vi "FPGA_Check_Pins_target.vi"() -> ()   [LabVIEW 2018]
uses:
  <vilib>/Platform/TimedLoop/XDataNode/timing_clust.ctl
  <vilib>/Platform/TimedLoop/XDataNode/nitl_modes.ctl
  <vilib>/Platform/TimedLoop/XDataNode/wakeup.ctl
  <vilib>/rvi/Emulation/niFpgaGetClockAttributes.vi
  <vilib>/rvi/Emulation/niFpgaSctlEmulationGetInTimedLoop.vi
  <vilib>/rvi/Emulation/niFpgaEmulationReportErrorSimple.vi
  <vilib>/rvi/eio/common/nirviEmuTemplateMethod_errors.vi
  <vilib>/rvi/Emulation/niFpgaCriticalErrorInLSC.vi
  <vilib>/rvi/Emulation/niFpgaProcessEmulError.vi
  <vilib>/eio/EIONode/EIONode.xnode
  <vilib>/Platform/TimedLoop/XDataNode/XDataNode.xnode
  <vilib>/Platform/TimedLoop/XDataNode/XDNodeRunTimeDep.lvlib
panel:
  out "Delay B to A":i16
  out "Delay A to B":i16
  out "Operation compl":bool
  out "DDCB_PFI3_Read":bool
  out "DDCB_PFI2_Read":bool
  out "DDCB_PFI1_Read":bool
  out "DDCA_PFI3_Read":bool
  out "DDCA_PFI2_Read":bool
  out "DDCA_PFI1_Read":bool
  in  "Write to PFI":u8
  in  "Cycle":bool
  out "Read Port 2 B":u8 format="%b"
  out "Read Port 1 B":u8 format="%b"
  out "Read Port 0 B":u8 format="%b"
  in  "A to B/B to A":bool
  in  "Write to":u8 format="%b"
  out "Read Port 2 A":u8 format="%b"
  out "Read Port 1 A":u8 format="%b"
  out "Read Port 0 A":u8 format="%b"
  in  "Source Freq":refnum<k21>="100 MHz Clock"
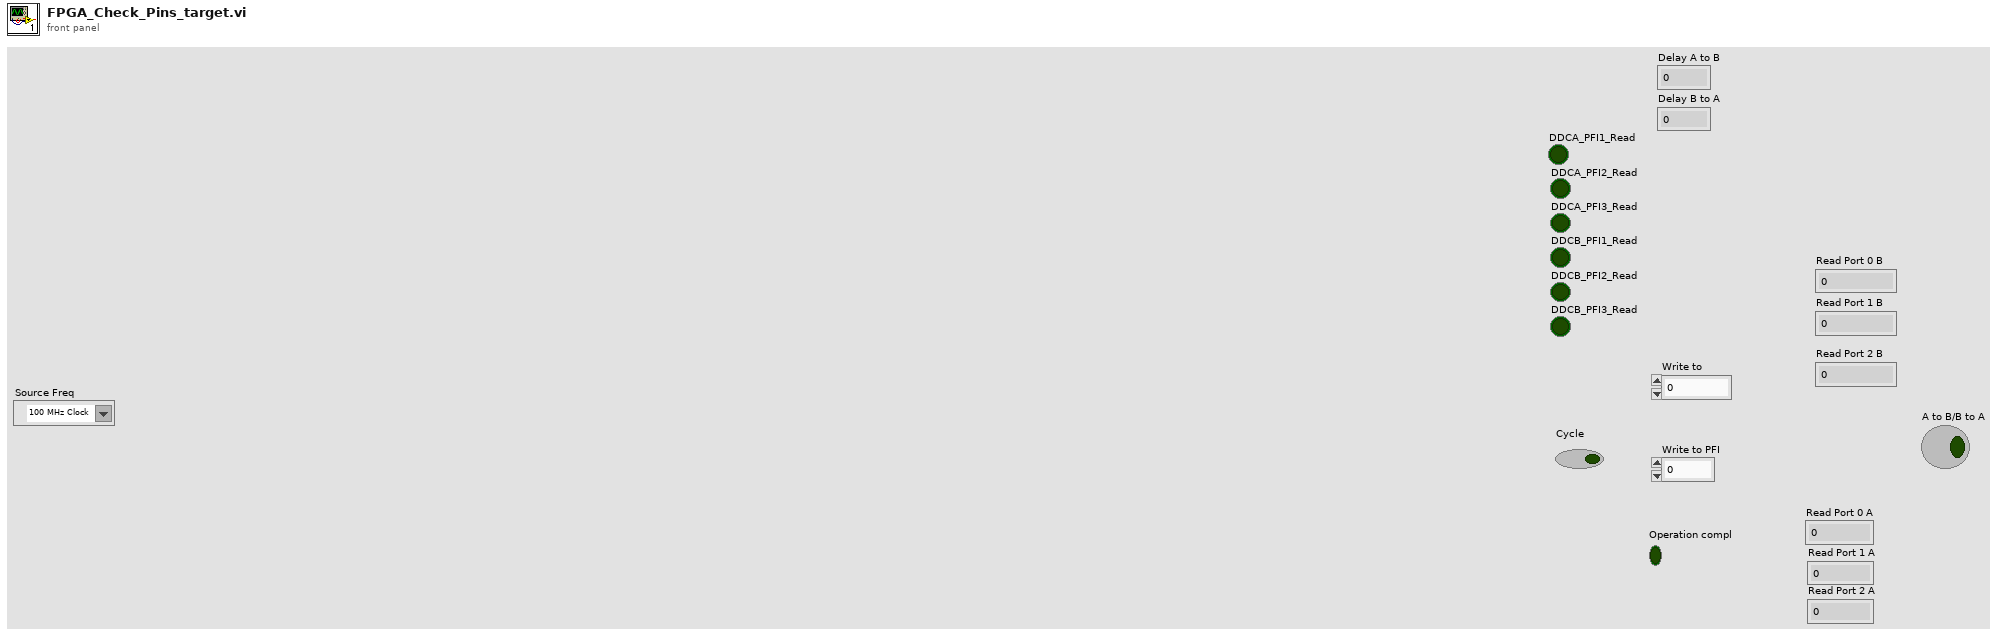
[diagram p1: front panel]
types:
  T1 = typedef "XDNodeRunTimeDep.lvlib/timing_clust.ctl" = cluster{"Expected End [f-1]":u64, "Actual End [f-1]":u64, "Finished Late? [f-1]":bool, "Expected End [i-1]":u64, "Actual End [i-1]":u64, "Finished Late? [i-1]":bool, "Expected Start [i]":u64, "Actual Start [i]":u64, "Expected Start [f]":u64, "Actual Start [f]":u64, "Source Name":string, "Structure Name":string, "Period":i64, "Deadline":i64, "Offset":i64, "Start":i64, "Priority":i32, "Timeout":i32, "Mode":T2, "Wakeup Reason":T3, "Error":errorcluster, "Source Type":string, "Secondary Source Type":string, "Global End Time":u64, "Global Start Time":u64, "Frame Duration":u64, "Iteration Duration":u64, "Assigned CPU":i32, "I/O Scan Engine Mode":u32}
  T2 = typedef "XDNodeRunTimeDep.lvlib/nitl_modes.ctl" = enum32{"No Change", "Process missed periods, maintain original phase", "Discard missed periods, maintain original phase", "Process missed periods, ignore original phase", "Discard missed periods, ignore original phase"}
  T3 = typedef "XDNodeRunTimeDep.lvlib/wakeup.ctl" = enum32{"Normal", "Aborted", "Asynchronous wakeup", "Timing source error", "Timed loop error", "Timeout"}
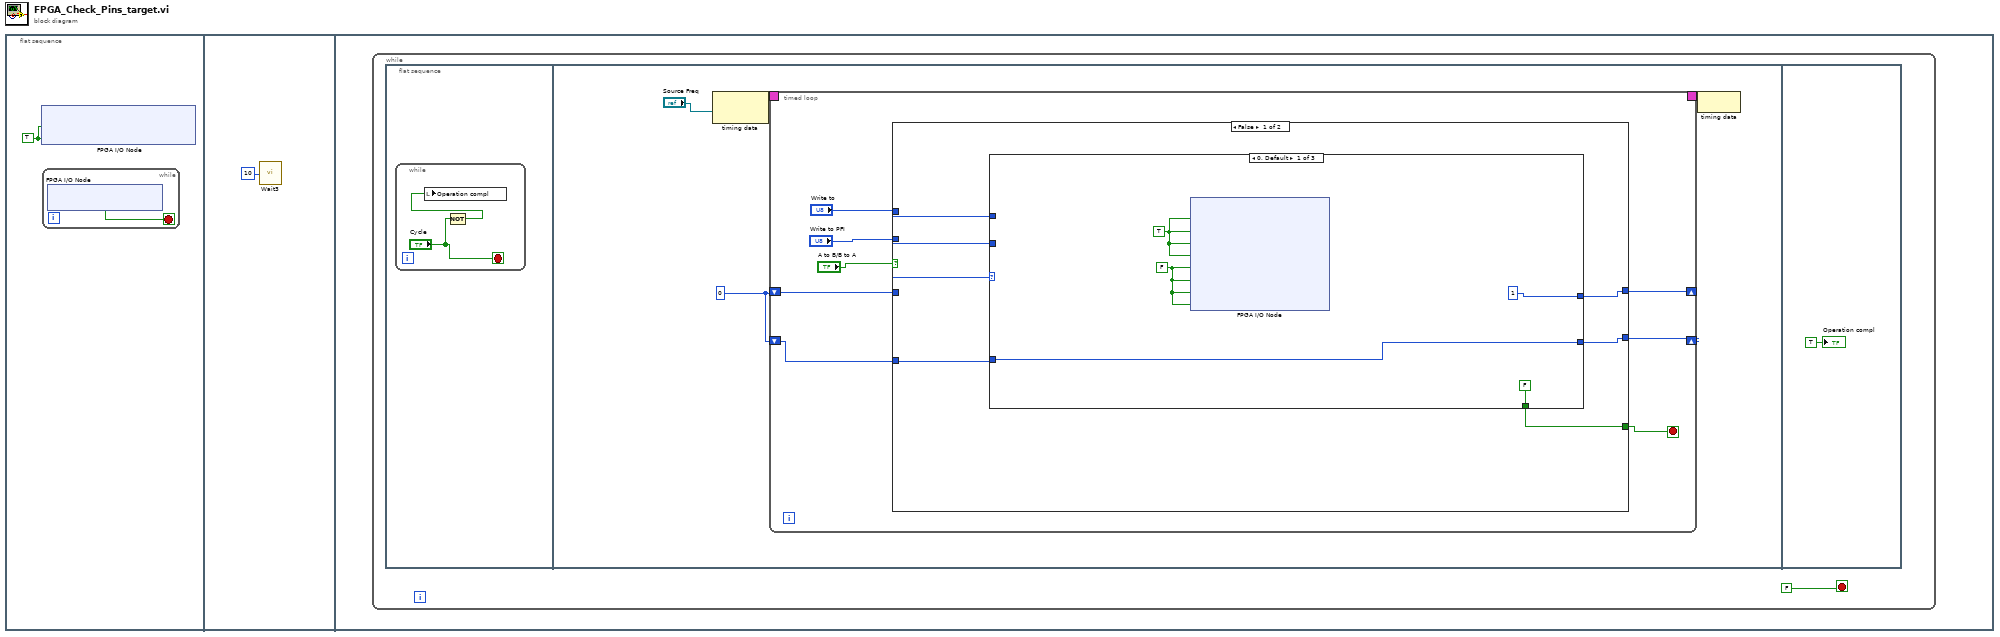
[diagram p0: block diagram]
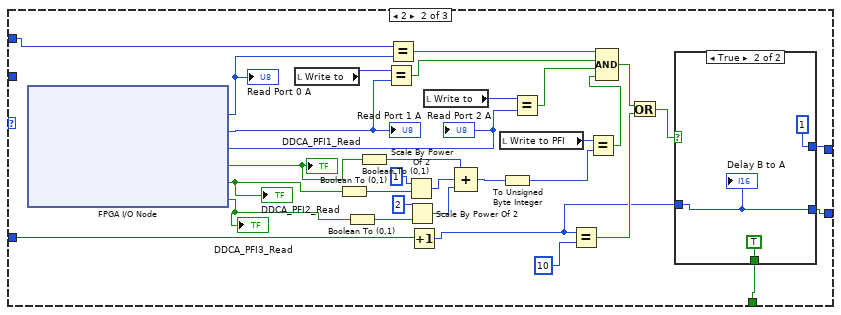
[diagram p2: hidden frame]
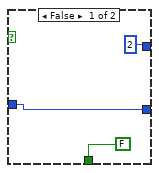
[diagram p3: hidden frame]
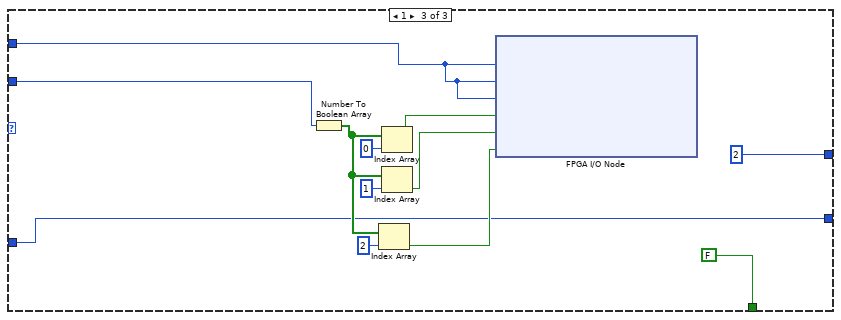
[diagram p4: hidden frame]
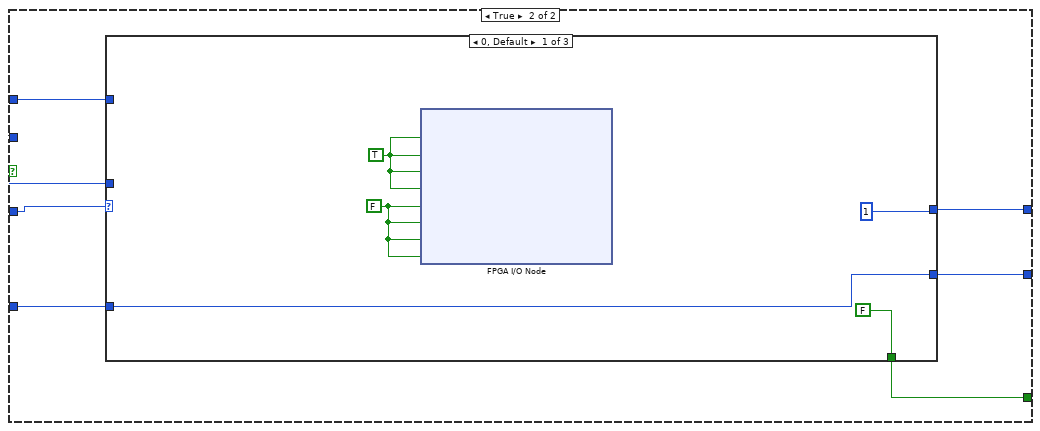
[diagram p5: hidden frame]
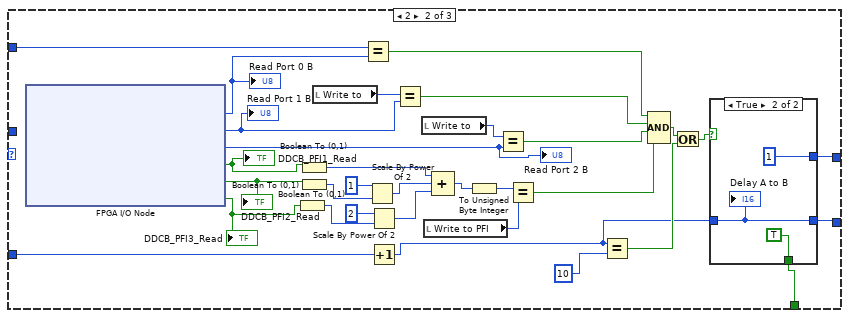
[diagram p6: hidden frame]
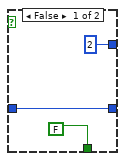
[diagram p7: hidden frame]
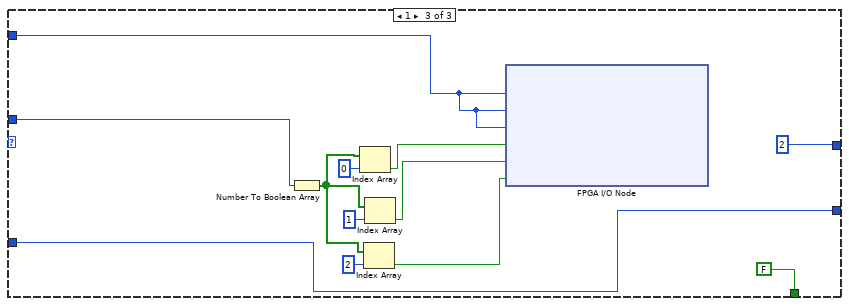
[diagram p8: hidden frame]
diagram:
  n1 = flat-sequence {
    frame #0 {
      w1 = TRUE ("IO Module\\DDCB_Supply_Select")
      n2 = xnode "FPGA I/O Node"("IO Module\\DDCB_Supply_Select"=w1, "IO Module\\DDCA_Supply_Select"=w1) -> ()  [unwired: 2 in, 2 out]
      n3 = while {
        stop <- w2 stop-if-true
        n4 = xnode "FPGA I/O Node"() -> ("IO Module IO Enabled"=w2:bool)  [unwired: 1 in, 1 out]
      }
    }
    frame #1 {
      n5 = call "Wait3"("Count(mSec)"=u8 10) -> ()  [unwired: 1 out]
    }
    frame #2 {
      n6 = while {
        stop <- FALSE stop-if-true
        n7 = flat-sequence {
          frame #0 {
            n8 = while {
              stop <- "Cycle" stop-if-true
              n9 = Not(x="Cycle") -> (.not. x?=w5:bool)
              n10 = local write "Operation compl"(w5) -> ()
            }
          }
          frame #1 {
            w7 = i16 0
            n11 = node-c288("Source Freq") -> (w10:T1)
            n12 = timed-loop {
              timing: w10 -> [_]
              timing-out: [_] -> w9
              shift-right: [w17] -> _
              shift-left: w7 -> [w18]
              shift-right: [w12] -> _
              shift-left: w7 -> [w11]
              stop <- w16 stop-if-true
              n13 = case shown="False" "A to B/B to A" {
                tunnel: w18 -> [w25 w87]
                tunnel: [w24 w86] -> w17
                tunnel: [w23 w85] -> w16
                tunnel: "Write to PFI" -> [w22 w84]
                tunnel: "Write to" -> [w21 w83]
                tunnel: [w19 w82] -> w12
                tunnel: w11 -> [w20 w81]
                frame False {
                  n14 = case shown="0, Default" w25 {
                    tunnel: [i16 1 w62 i16 2] -> w24
                    tunnel: [FALSE w61 FALSE] -> w23
                    tunnel: w22 -> [_ _ w71]
                    tunnel: w21 -> [_ w47 w70]
                    tunnel: w20 -> [w28 w54 w69]
                    tunnel: [w28 w48 w69] -> w19
                    frame 0, Default {
                      w26 = FALSE ("IO Module\\DDCA_Port0_WE")
                      w30 = TRUE
                      n15 = xnode "FPGA I/O Node"("IO Module\\DDCB_Port0_WE"=w30, "IO Module\\DDCB_Port1_WE"=w30, "IO Module\\DDCB_Port2_WE"=w30, "IO Module\\DDCB_PFI_WE"=w30, "IO Module\\DDCA_Port0_WE"=w26, "IO Module\\DDCA_Port1_WE"=w26, "IO Module\\DDCA_Port2_WE"=w26, "IO Module\\DDCA_PFI_WE"=w26) -> ()  [unwired: 8 in, 8 out]
                    }
                    frame 2 {
                      n16 = xnode "FPGA I/O Node"() -> ("IO Module\\DDCA_Port0_Read"=w59:u8, "IO Module\\DDCA_Port1_Read"=w57:u8, "IO Module\\DDCA_Port2_Read"=w56:u8, "IO Module\\DDCA_PFI1_Read"=w44:bool, "IO Module\\DDCA_PFI2_Read"=w42:bool, "IO Module\\DDCA_PFI3_Read"=w43:bool)  [unwired: 6 in, 6 out]
                      "Read Port 0 A" <- w59
                      "Read Port 1 A" <- w57
                      "Read Port 2 A" <- w56
                      "DDCA_PFI1_Read" <- w44
                      "DDCA_PFI2_Read" <- w42
                      "DDCA_PFI3_Read" <- w43
                      n17 = local read "Write to"() -> (w46:u8)
                      n18 = Boolean To (0,1)(Boolean=w42) -> (0, 1=w38:i16)
                      n19 = Boolean To (0,1)(Boolean=w43) -> (0, 1=w35:i16)
                      n20 = Boolean To (0,1)(Boolean=w44) -> (0, 1=w41:i16)
                      n21 = Equal?(x=w46, y=w57) -> (x = y?=w58:bool)
                      n22 = Equal?(x=w47, y=w59) -> (x = y?=w60:bool)
                      n23 = Scale By Power Of 2(n=i16 1, x=w38) -> (x*2^n=w36:i16)
                      n24 = Scale By Power Of 2(n=i16 2, x=w35) -> (x*2^n=w33:i16)
                      n25 = Increment(x=w54) -> (x+1=w49:i16)
                      n26 = local read "Write to"() -> (w45:u8)
                      n27 = Compound Arithmetic op=unknown(w41, w36, w33) -> (w31:i16)
                      n28 = local read "Write to PFI"() -> (w40:u8)
                      n29 = To Unsigned Byte Integer(number=w31) -> (unsigned 8bit integer=w32:u8)
                      n30 = Equal?(x=w45, y=w56) -> (x = y?=w55:bool)
                      n31 = Equal?(x=w49, y=i16 10) -> (x = y?=w51:bool)
                      n32 = Equal?(x=w40, y=w32) -> (x = y?=w39:bool)
                      n33 = Compound Arithmetic op=AND(w60, w58, w55, w39) -> (w52:bool)
                      n34 = Or(x=w52, y=w51) -> (x .or. y?=w50:bool)
                      n35 = case shown="True" w50 {
                        tunnel: [i16 2 i16 1] -> w62
                        tunnel: [FALSE TRUE] -> w61
                        tunnel: w49 -> [w63 w66]
                        tunnel: [w63 w66] -> w48
                        frame False {
                        }
                        frame True {
                          "Delay B to A" <- w66
                        }
                      }
                    }
                    frame 1 {
                      n36 = Number To Boolean Array(number=w71) -> (Boolean array=w78:bool[])
                      n37 = Index Array(array=w78, index=2) -> (element=w72:bool)
                      n38 = Index Array(array=w78, index=0) -> (element=w74:bool)
                      n39 = Index Array(array=w78, index=1) -> (element=w73:bool)
                      n40 = xnode "FPGA I/O Node"("IO Module\\DDCB_Port0_Write"=w70, "IO Module\\DDCB_Port1_Write"=w70, "IO Module\\DDCB_Port2_Write"=w70, "IO Module\\DDCB_PFI1_Write"=w74, "IO Module\\DDCB_PFI2_Write"=w73, "IO Module\\DDCB_PFI3_Write"=w72) -> ()  [unwired: 6 in, 6 out]
                    }
                  }
                }
                frame True {
                  n41 = case shown="0, Default" w87 {
                    tunnel: [i16 1 w124 i16 2] -> w86
                    tunnel: [FALSE w123 FALSE] -> w85
                    tunnel: w84 -> [_ _ w133]
                    tunnel: w83 -> [_ w119 w132]
                    tunnel: [w90 w109 w131] -> w82
                    tunnel: w81 -> [w90 w122 w131]
                    frame 0, Default {
                      w88 = FALSE ("IO Module\\DDCB_Port0_WE")
                      w92 = TRUE
                      n42 = xnode "FPGA I/O Node"("IO Module\\DDCA_Port0_WE"=w92, "IO Module\\DDCA_Port1_WE"=w92, "IO Module\\DDCA_Port2_WE"=w92, "IO Module\\DDCA_PFI_WE"=w92, "IO Module\\DDCB_Port0_WE"=w88, "IO Module\\DDCB_Port1_WE"=w88, "IO Module\\DDCB_Port2_WE"=w88, "IO Module\\DDCB_PFI_WE"=w88) -> ()  [unwired: 8 in, 8 out]
                    }
                    frame 2 {
                      n43 = xnode "FPGA I/O Node"() -> ("IO Module\\DDCB_Port0_Read"=w121:u8, "IO Module\\DDCB_Port1_Read"=w117:u8, "IO Module\\DDCB_Port2_Read"=w118:u8, "IO Module\\DDCB_PFI1_Read"=w104:bool, "IO Module\\DDCB_PFI2_Read"=w105:bool, "IO Module\\DDCB_PFI3_Read"=w106:bool)  [unwired: 6 in, 6 out]
                      "Read Port 0 B" <- w121
                      "Read Port 1 B" <- w117
                      "Read Port 2 B" <- w118
                      "DDCB_PFI1_Read" <- w104
                      "DDCB_PFI2_Read" <- w105
                      "DDCB_PFI3_Read" <- w106
                      n44 = Boolean To (0,1)(Boolean=w106) -> (0, 1=w96:i16)
                      n45 = Boolean To (0,1)(Boolean=w104) -> (0, 1=w93:i16)
                      n46 = Boolean To (0,1)(Boolean=w105) -> (0, 1=w97:i16)
                      n47 = local read "Write to"() -> (w108:u8)
                      n48 = Equal?(x=w119, y=w121) -> (x = y?=w120:bool)
                      n49 = Scale By Power Of 2(n=i16 1, x=w97) -> (x*2^n=w99:i16)
                      n50 = Scale By Power Of 2(n=i16 2, x=w96) -> (x*2^n=w98:i16)
                      n51 = Increment(x=w122) -> (x+1=w110:i16)
                      n52 = Equal?(x=w108, y=w117) -> (x = y?=w116:bool)
                      n53 = local read "Write to"() -> (w107:u8)
                      n54 = local read "Write to PFI"() -> (w103:u8)
                      n55 = Compound Arithmetic op=unknown(w93, w99, w98) -> (w102:i16)
                      n56 = To Unsigned Byte Integer(number=w102) -> (unsigned 8bit integer=w101:u8)
                      n57 = Equal?(x=w107, y=w118) -> (x = y?=w115:bool)
                      n58 = Equal?(x=w101, y=w103) -> (x = y?=w100:bool)
                      n59 = Equal?(x=w110, y=i16 10) -> (x = y?=w112:bool)
                      n60 = Compound Arithmetic op=AND(w120, w116, w115, w100) -> (w114:bool)
                      n61 = Or(x=w114, y=w112) -> (x .or. y?=w113:bool)
                      n62 = case shown="True" w113 {
                        tunnel: [i16 2 i16 1] -> w124
                        tunnel: [FALSE TRUE] -> w123
                        tunnel: [w125 w128] -> w109
                        tunnel: w110 -> [w125 w128]
                        frame False {
                        }
                        frame True {
                          "Delay A to B" <- w128
                        }
                      }
                    }
                    frame 1 {
                      n63 = Number To Boolean Array(number=w133) -> (Boolean array=w139:bool[])
                      n64 = Index Array(array=w139, index=0) -> (element=w140:bool)
                      n65 = Index Array(array=w139, index=2) -> (element=w134:bool)
                      n66 = Index Array(array=w139, index=1) -> (element=w135:bool)
                      n67 = xnode "FPGA I/O Node"("IO Module\\DDCA_Port0_Write"=w132, "IO Module\\DDCA_Port1_Write"=w132, "IO Module\\DDCA_Port2_Write"=w132, "IO Module\\DDCA_PFI1_Write"=w140, "IO Module\\DDCA_PFI2_Write"=w135, "IO Module\\DDCA_PFI3_Write"=w134) -> ()  [unwired: 6 in, 6 out]
                    }
                  }
                }
              }
            }
            n68 = node-c288(w9) -> ()
          }
          frame #2 {
            "Operation compl" <- TRUE ("Boolean")
          }
        }
      }
    }
  }
